vi "Swerve Drive.vi"(8 "error in":errorcluster) -> ()   [LabVIEW 2018]
doc: "This VI runs in parallel to other tasks. It can contain as many user-defined periodic loops as you need. These can carry out PID or other sorts of timed response."
uses:
  <vilib>/Rock Robotics/WPI/ThirdParty/Phoenix-LabVIEW/Motor Controller/Controls/CTRE_Phoenix_MotorControl_ControlMode.ctl
  navx-mxp/labview/navX Library v2/navX Library v2.lvlib
panel:
  in  "Rewrite Offsets":bool
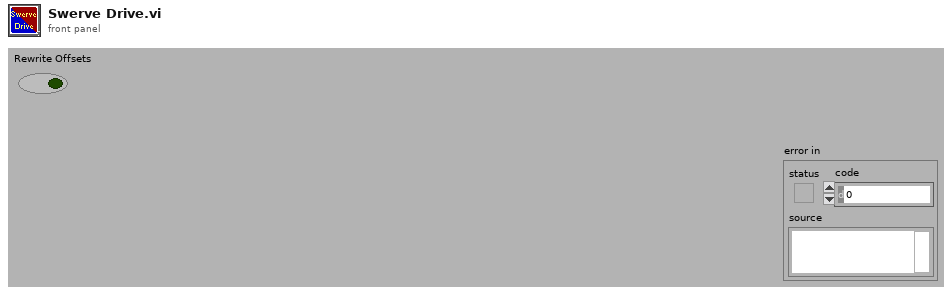
[diagram p1: front panel]
types:
  T1 = typedef "WPI_AnalogChannelDevRef.ctl" = cluster{"DevStatus":errorcluster, "Analog Channel":T2}
  T2 = typedef "FPGA_AIChannel.ctl" = enum8{"AI 0", "AI 1", "AI 2", "AI 3", "AI MXP 0", "AI MXP 1", "AI MXP 2", "AI MXP 3", "Invalid"}
  T3 = typedef "navX Library v2.lvlib/Z900_navX_DeviceTypeDef.ctl" = cluster{"Interface":cluster{"Protocol":T4, "Update Rate (4Hz-100Hz)":u8, "navX Open TypeDef":variant}, "Notify Packet":refnum<notifier>, "Loop VI Refnum":refnum<vi>, "Ready to Close Occurrence Refnum":refnum<k4>}
  T4 = typedef "navX Library v2.lvlib/Z900_navX_ProtocolTypeDef.ctl" = enum16{"SERIAL", "I2C", "SPI"}
  T5 = typedef "WPI_JoystickDevRef.ctl" = cluster{"Device":T6}
  T6 = typedef "WPI_JoystickDeviceEnum.ctl" = enum16{"USB 0", "USB 1", "USB 2", "USB 3", "USB 4", "USB 5"}
  T7 = typedef "WPI_MotorControlDeviceRef.ctl" = cluster{"DeviceStatus":errorcluster, "Type":T8, "PWM":cluster{"PWM Channel":T9, "DeadBand":T10}, "CAN":cluster{"Device Number":u8, "SetOutput VI Ref":variant, "GetOutput VI Ref":variant, "Enable VI Ref":variant, "Disable VI Ref":variant, "Data":variant}, "Invert":bool, "DIO PWM":cluster{"PWM \"Enable\" Channel":T9, "DIOChannel":T11, "PWM Rate":dbl}}
  T8 = typedef "WPI_MotorControlType.ctl" = enum16{"PWM", "CAN", "DIO PWM"}
  T9 = typedef "FPGA_DIOPWMChannel.ctl" = enum8{"PWM 0", "PWM 1", "PWM 2", "PWM 3", "PWM 4", "PWM 5", "PWM 6", "PWM 7", "PWM 8", "PWM 9", "PWM MXP 0", "PWM MXP 1", "PWM MXP 2", "PWM MXP 3", "PWM MXP 4", "PWM MXP 5", "PWM MXP 6", "PWM MXP 7", "PWM MXP 8", "PWM MXP 9", "Invalid"}
  T10 = typedef "WPI_PWMDeadband.ctl" = cluster{"Name":string, "maxPositivePwm":i32, "minPositivePwm":i32, "centerPwm":i32, "maxNegativePwm":i32, "minNegativePwm":i32, "angularRange":u16}
  T11 = typedef "FPGA_DIOChannel.ctl" = enum8{"DIO 0", "DIO 1", "DIO 2", "DIO 3", "DIO 4", "DIO 5", "DIO 6", "DIO 7", "DIO 8", "DIO 9", "DIO MXP 0", "DIO MXP 1", "DIO MXP 2", "DIO MXP 3", "DIO MXP 4", "DIO MXP 5", "DIO MXP 6", "DIO MXP 7", "DIO MXP 8", "DIO MXP 9", "DIO MXP 10", "DIO MXP 11", "DIO MXP 12", "DIO MXP 13", "DIO MXP 14", "DIO MXP 15", "SPI Port CS1", "SPI Port CS2", "SPI Port CS3", "SPI Port MISO", "SPI Port MOSI", "Invalid"}
  T12 = cluster{"PhoenixMotorControlDevRef":T7, "PhoenixMotorControlDevRef":T7, "PhoenixMotorControlDevRef":T7, "PhoenixMotorControlDevRef":T7}
  T13 = typedef "CTRE_Phoenix_MotorControl_ControlMode.ctl" = u16
  T14 = cluster{"Yaw":dbl, "Roll":dbl, "Pitch":dbl, "Heading":dbl, "Fused Heading":dbl}
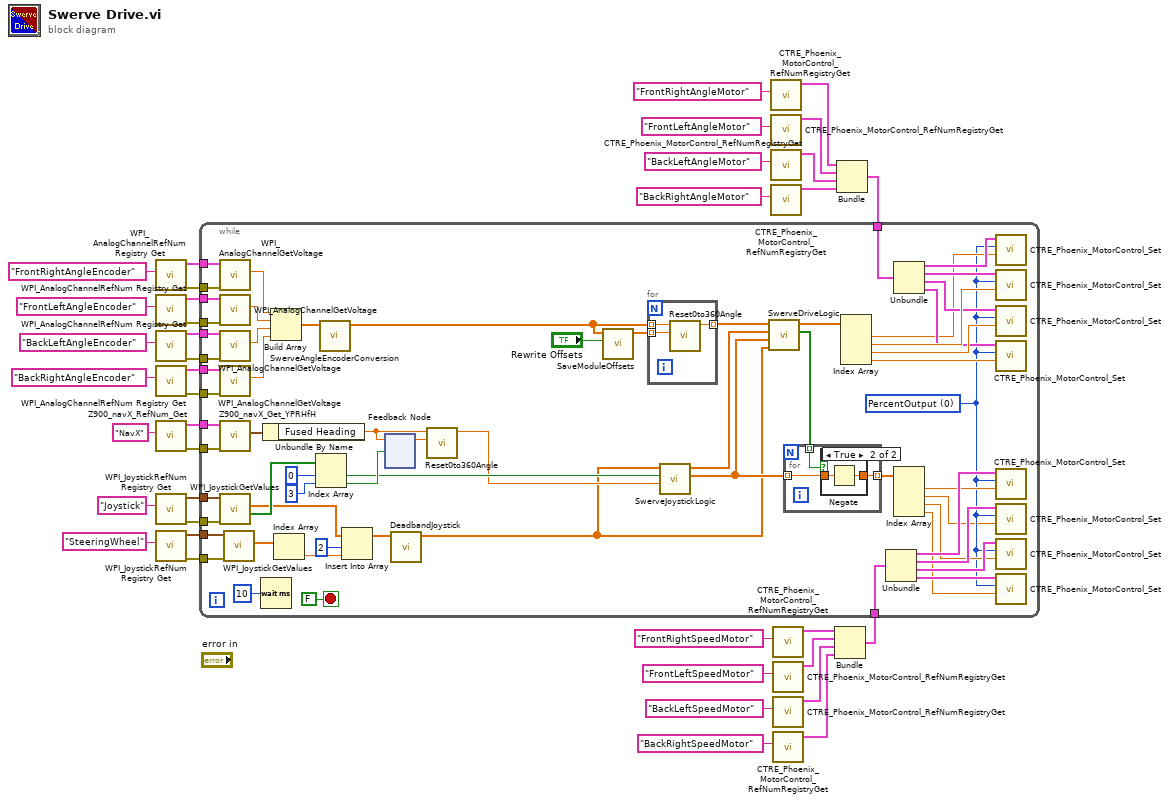
[diagram p0: block diagram]
diagram:
  n1 = call <vilib>:"WPI_AnalogChannelRefNum Registry Get.vi"("refnum name"="FrontRightAngleEncoder") -> ("error out"=w15:errorcluster, "AIDeviceRef"=w25:T1)  [unwired: 9 in]
  n2 = call <vilib>:"WPI_AnalogChannelRefNum Registry Get.vi"("refnum name"="FrontLeftAngleEncoder") -> ("error out"=w14:errorcluster, "AIDeviceRef"=w24:T1)  [unwired: 9 in]
  n3 = call <vilib>:"WPI_AnalogChannelRefNum Registry Get.vi"("refnum name"="BackLeftAngleEncoder") -> ("error out"=w13:errorcluster, "AIDeviceRef"=w23:T1)  [unwired: 9 in]
  n4 = call <vilib>:"WPI_AnalogChannelRefNum Registry Get.vi"("refnum name"="BackRightAngleEncoder") -> ("error out"=w12:errorcluster, "AIDeviceRef"=w22:T1)  [unwired: 9 in]
  n5 = call "Z900_navX_RefNum_Get.vi"("refnum name"="NavX") -> ("error out"=w10:errorcluster, "navX Device"=w11:T3)  [unwired: 9 in]
  n6 = call <vilib>:"WPI_JoystickRefNum Registry Get.vi"("refnum name"="Joystick") -> ("error out"=w4:errorcluster, "JoystickDevRef"=w5:T5)  [unwired: 1 in, 8 out]
  n7 = call <vilib>:"WPI_JoystickRefNum Registry Get.vi"("refnum name"="SteeringWheel") -> ("error out"=w2:errorcluster, "JoystickDevRef"=w3:T5)  [unwired: 1 in, 8 out]
  n8 = call <vilib>:"CTRE_Phoenix_MotorControl_RefNumRegistryGet.vi"("refnum name"="FrontRightAngleMotor") -> ("PhoenixMotorControlDevRef"=w16:T7)  [unwired: 9 in, 1 out]
  n9 = call <vilib>:"CTRE_Phoenix_MotorControl_RefNumRegistryGet.vi"("refnum name"="FrontLeftAngleMotor") -> ("PhoenixMotorControlDevRef"=w20:T7)  [unwired: 9 in, 1 out]
  n10 = call <vilib>:"CTRE_Phoenix_MotorControl_RefNumRegistryGet.vi"("refnum name"="BackLeftAngleMotor") -> ("PhoenixMotorControlDevRef"=w21:T7)  [unwired: 9 in, 1 out]
  n11 = call <vilib>:"CTRE_Phoenix_MotorControl_RefNumRegistryGet.vi"("refnum name"="BackRightAngleMotor") -> ("PhoenixMotorControlDevRef"=w18:T7)  [unwired: 9 in, 1 out]
  n12 = call <vilib>:"CTRE_Phoenix_MotorControl_RefNumRegistryGet.vi"("refnum name"="FrontRightSpeedMotor") -> ("PhoenixMotorControlDevRef"=w19:T7)  [unwired: 9 in, 1 out]
  n13 = call <vilib>:"CTRE_Phoenix_MotorControl_RefNumRegistryGet.vi"("refnum name"="FrontLeftSpeedMotor") -> ("PhoenixMotorControlDevRef"=w1:T7)  [unwired: 9 in, 1 out]
  n14 = call <vilib>:"CTRE_Phoenix_MotorControl_RefNumRegistryGet.vi"("refnum name"="BackLeftSpeedMotor") -> ("PhoenixMotorControlDevRef"=w26:T7)  [unwired: 9 in, 1 out]
  n15 = call <vilib>:"CTRE_Phoenix_MotorControl_RefNumRegistryGet.vi"("refnum name"="BackRightSpeedMotor") -> ("PhoenixMotorControlDevRef"=w27:T7)  [unwired: 9 in, 1 out]
  n16 = Bundle("PhoenixMotorControlDevRef"=w19, "PhoenixMotorControlDevRef"=w1, "PhoenixMotorControlDevRef"=w26, "PhoenixMotorControlDevRef"=w27) -> (w8:T12)  [unwired: 1 in]
  n17 = Bundle("PhoenixMotorControlDevRef"=w16, "PhoenixMotorControlDevRef"=w20, "PhoenixMotorControlDevRef"=w21, "PhoenixMotorControlDevRef"=w18) -> (w17:T12)  [unwired: 1 in]
  n18 = while {
    tunnel: w25 -> [w77]
    tunnel: w24 -> [w72]
    tunnel: w23 -> [w69]
    tunnel: w22 -> [w75]
    tunnel: w17 -> [w85]
    tunnel: w15 -> [w78]
    tunnel: w14 -> [w71]
    tunnel: w13 -> [w68]
    tunnel: w12 -> [w74]
    tunnel: w11 -> [w62]
    tunnel: w10 -> [w61]
    tunnel: w8 -> [w57]
    tunnel: w5 -> [w49]
    tunnel: w4 -> [w48]
    tunnel: w3 -> [w45]
    tunnel: w2 -> [w44]
    stop <- FALSE stop-if-true
    w79 = T13 0 items=["PercentOutput"=0, "Position"=1, "Velocity"=2, "Current"=3, "Follower"=5, "MotionProfile"=6, "MotionMagic"=7, "MotionProfileArc"=10, "Disabled"=15] ("Control Mode")
    n19 = call <vilib>:"WPI_AnalogChannelGetVoltage.vi"("error in (no error)"=w78, "AIDeviceRef"=w77) -> ("Voltage"=w76:dbl)  [unwired: 7 in, 2 out]
    n20 = call <vilib>:"WPI_AnalogChannelGetVoltage.vi"("error in (no error)"=w71, "AIDeviceRef"=w72) -> ("Voltage"=w70:dbl)  [unwired: 7 in, 2 out]
    n21 = call <vilib>:"WPI_AnalogChannelGetVoltage.vi"("error in (no error)"=w68, "AIDeviceRef"=w69) -> ("Voltage"=w67:dbl)  [unwired: 7 in, 2 out]
    n22 = call <vilib>:"WPI_AnalogChannelGetVoltage.vi"("error in (no error)"=w74, "AIDeviceRef"=w75) -> ("Voltage"=w73:dbl)  [unwired: 7 in, 2 out]
    n23 = call "Z900_navX_Get_YPRHfH.vi"("error in (no error)"=w61, "navX Device"=w62) -> ("YRPHfH"=w63:T14)  [unwired: 6 in, 3 out]
    n24 = call <vilib>:"WPI_JoystickGetValues.vi"("error in (no error)"=w48, "JoystickDevRef"=w49) -> ("Buttons"=w54:bool[], "Axes"=w42:dbl[])  [unwired: 5 in, 3 out]
    n25 = call <vilib>:"WPI_JoystickGetValues.vi"("error in (no error)"=w44, "JoystickDevRef"=w45) -> ("Axes"=w53:dbl[])  [unwired: 5 in, 4 out]
    n26 = Wait (ms)(milliseconds to wait=u32 10) -> ()  [unwired: 1 out]
    n27 = Unbundle By Name(w63) -> ("Fused Heading"=w47:dbl)
    n28 = Build Array(w76, w70, w67, w73) -> (w84:dbl[])
    n29 = Index Array(array=w53) -> (element=w56:dbl)  [unwired: 1 in]
    n30 = Index Array(array=w54, index #1=0 ("index"), index #2=3 ("index")) -> (element #1=w43:bool, element #2=w46:bool)
    n31 = call "SwerveAngleEncoderConversion.vi"("Voltages"=w84) -> ("Angles"=w59:dbl[])  [unwired: 10 in]
    n32 = Insert Into Array(array=w42, index=2, new element=w56) -> (w55:dbl[])
    n33 = feedback #1() -> (w64:dbl)  [unwired: 1 in]
    n34 = feedback-in #1(w47, w46) -> ()
    n35 = call "DeadbandJoystick.vi"("InputArray"=w55) -> ("OutputArray"=w40:dbl[])  [unwired: 10 in]
    n36 = call "Reset0to360Angle.vi"("Offset"=w64, "AngleInput"=w47) -> ("AngleOutput"=w41:dbl)  [unwired: 9 in]
    n37 = call "SaveModuleOffsets.vi"("Write Swerve Offsets"="Rewrite Offsets", "Swerve Voltages"=w59) -> ("Swerve Offsets"=w60:dbl[])  [unwired: 9 in]
    n38 = for {
      tunnel: w59 -> [w105] mode=indexing
      tunnel: [w106] -> w91 mode=indexing
      tunnel: w60 -> [w104] mode=indexing
      n39 = call "Reset0to360Angle.vi"("Offset"=w104, "AngleInput"=w105) -> ("AngleOutput"=w106:dbl)  [unwired: 9 in]
    }
    n40 = call "SwerveJoystickLogic.vi"("Gyro"=w41, "Ackerman"=w43, "Joystick Axes"=w40) -> ("Speeds"=w88:dbl[], "Angles"=w90:dbl[])  [unwired: 6 in]
    n41 = call "SwerveDriveLogic.vi"("Joystick Axes"=w40, "Speeds"=w88, "AngleSetpoints"=w90, "AngleEncoders"=w91) -> ("AngleMotorsReversed"=w92:bool[], "AngleMotorOutputs"=w89:dbl[])  [unwired: 6 in]
    n42 = for {
      tunnel: w88 -> [w108] mode=indexing
      tunnel: [w109] -> w97 mode=indexing
      tunnel: w92 -> [w107] mode=indexing
      n43 = case shown="True" w107 {
        tunnel: w108 -> [w110 w112]
        tunnel: [w110 w111] -> w109
        frame False {
        }
        frame True {
          n44 = Negate(x=w112) -> (-x=w111:dbl)
        }
      }
    }
    n45 = Index Array(array=w89) -> (element #1=w82:dbl, element #2=w102:dbl, element #3=w101:dbl, element #4=w83:dbl)  [unwired: 4 in]
    n46 = Unbundle(w57) -> ("PhoenixMotorControlDevRef"=w87:T7, "PhoenixMotorControlDevRef"=w96:T7, "PhoenixMotorControlDevRef"=w95:T7, "PhoenixMotorControlDevRef"=w94:T7)
    n47 = Unbundle(w85) -> ("PhoenixMotorControlDevRef"=w100:T7, "PhoenixMotorControlDevRef"=w99:T7, "PhoenixMotorControlDevRef"=w98:T7, "PhoenixMotorControlDevRef"=w93:T7)
    n48 = Index Array(array=w97) -> (element #1=w81:dbl, element #2=w65:dbl, element #3=w80:dbl, element #4=w66:dbl)  [unwired: 4 in]
    n49 = call <vilib>:"CTRE_Phoenix_MotorControl_Set.vi"("Output"=w82, "Control Mode"=w79, "PhoenixMotorControlDevRef"=w100) -> ()  [unwired: 7 in, 2 out]
    n50 = call <vilib>:"CTRE_Phoenix_MotorControl_Set.vi"("Output"=w102, "Control Mode"=w79, "PhoenixMotorControlDevRef"=w99) -> ()  [unwired: 7 in, 2 out]
    n51 = call <vilib>:"CTRE_Phoenix_MotorControl_Set.vi"("Output"=w101, "Control Mode"=w79, "PhoenixMotorControlDevRef"=w98) -> ()  [unwired: 7 in, 2 out]
    n52 = call <vilib>:"CTRE_Phoenix_MotorControl_Set.vi"("Output"=w83, "Control Mode"=w79, "PhoenixMotorControlDevRef"=w93) -> ()  [unwired: 7 in, 2 out]
    n53 = call <vilib>:"CTRE_Phoenix_MotorControl_Set.vi"("Output"=w81, "Control Mode"=w79, "PhoenixMotorControlDevRef"=w87) -> ()  [unwired: 7 in, 2 out]
    n54 = call <vilib>:"CTRE_Phoenix_MotorControl_Set.vi"("Output"=w65, "Control Mode"=w79, "PhoenixMotorControlDevRef"=w96) -> ()  [unwired: 7 in, 2 out]
    n55 = call <vilib>:"CTRE_Phoenix_MotorControl_Set.vi"("Output"=w80, "Control Mode"=w79, "PhoenixMotorControlDevRef"=w95) -> ()  [unwired: 7 in, 2 out]
    n56 = call <vilib>:"CTRE_Phoenix_MotorControl_Set.vi"("Output"=w66, "Control Mode"=w79, "PhoenixMotorControlDevRef"=w94) -> ()  [unwired: 7 in, 2 out]
  }
